vi "isComplete.vi"(8 "error in (no error)":errorcluster, 11 "Mission in":refnum<class "GenericMission.lvclass">) -> (0 "error out":errorcluster, 2 "Mission Complete?":bool, 3 "Mission out":refnum<class "GenericMission.lvclass">)   [LabVIEW 2011, in "GenericMission.lvclass"]
doc: "Determine whether or not a mission is complete.\n\nImplementation note: this may need to take sensorData.ctl as an input.\n\nAuthor: Jared Kirschner"
uses:
  GenericMission.lvclass
  2 Globals/2 Global.vi
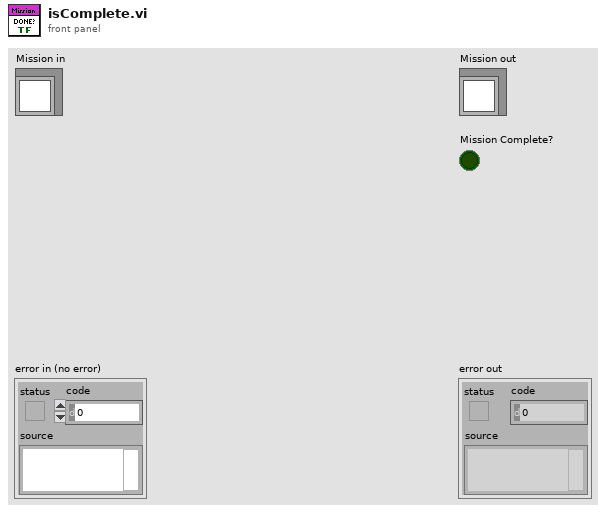
[diagram p1: front panel]
types:
  T1 = typedef "Current Waypoint.ctl" = i32
  T2 = typedef "Waypoints List.ctl" = refnum<class "Waypoint.lvclass">[]
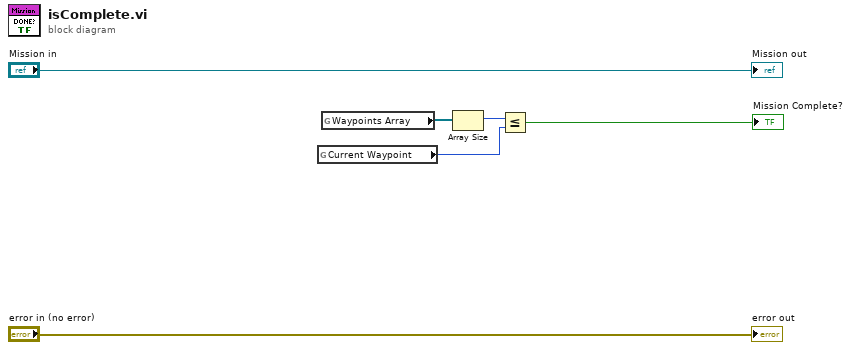
[diagram p0: block diagram]
diagram:
  n1 = global read "2 Global.vi" "Current Waypoint"() -> (w1:T1)
  n2 = global read "2 Global.vi" "Waypoints Array"() -> (w3:T2)
  n3 = Array Size(array=w3) -> (size(s)=w2:i32)
  n4 = Less Or Equal?(x=w2, y=w1) -> (x <= y?=→"Mission Complete?":bool)
  "error out" <- "error in (no error)"
  "Mission out" <- "Mission in"
